vi "Set Protocol Switch Threshold.vi"(8 "error in":errorcluster, 10 "Protocol Switch Threshold":u8, 11 "Block Upload Initiate in":refnum<class "Block Upload Initiate Transfer.lvclass">) -> (0 "error out":errorcluster, 3 "Block Upload Initiate out":refnum<class "Block Upload Initiate Transfer.lvclass">)   [LabVIEW 2020, in "CANopen.lvlib" / "SDO Manager.lvlib" / "Block Upload Initiate Transfer.lvclass"]
uses:
  Block Upload Initiate Transfer.lvclass
  Block Upload Initiate Transfer.lvclass/Block Upload Initiate Transfer.ctl
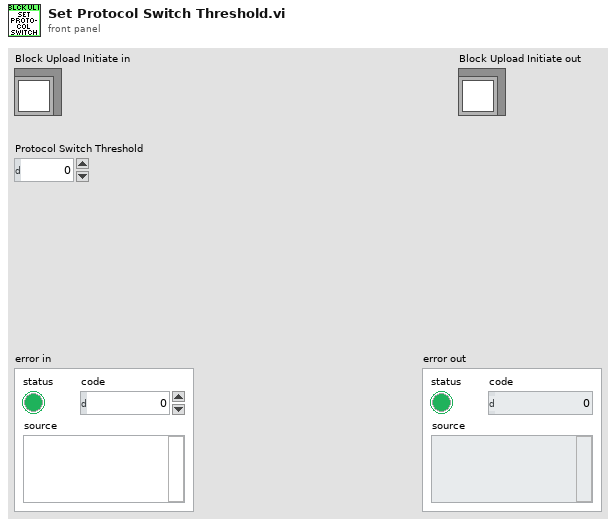
[diagram p1: front panel]
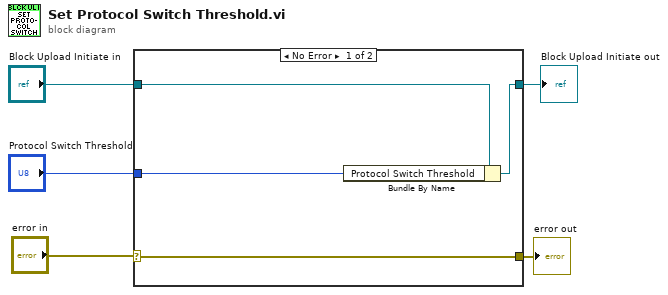
[diagram p0: block diagram]
diagram:
  n1 = case shown="No Error" "error in" {
    selector: "error in" -> [w9 w10]
    tunnel: [w9 w10] -> w2
    tunnel: [w7 w11] -> w4
    tunnel: "Block Upload Initiate in" -> [w8 w11]
    tunnel: "Protocol Switch Threshold" -> [w6 _]
    frame No Error {
      n2 = Bundle By Name(cluster=w8, "Protocol Switch Threshold"=w6) -> (w7:refnum<class "Block Upload Initiate Transfer.lvclass">)
    }
    frame Error {
    }
  }
  "error out" <- w2
  "Block Upload Initiate out" <- w4
